vi "split.vi"(0 "object in":refnum<class "access_work.lvclass">, 1 "输入数据":string[][](array[string]), 2 "拆分大小":i32=1000, 5 "error in (no error)":errorcluster) -> (14 "object out":refnum<class "access_work.lvclass">, 15 "输出数组":string[][](array[string]), 16 "拆分数据":bool, 19 "error out":errorcluster)   [LabVIEW 2016, in "access_work.lvclass"]
uses:
  access_work.lvclass
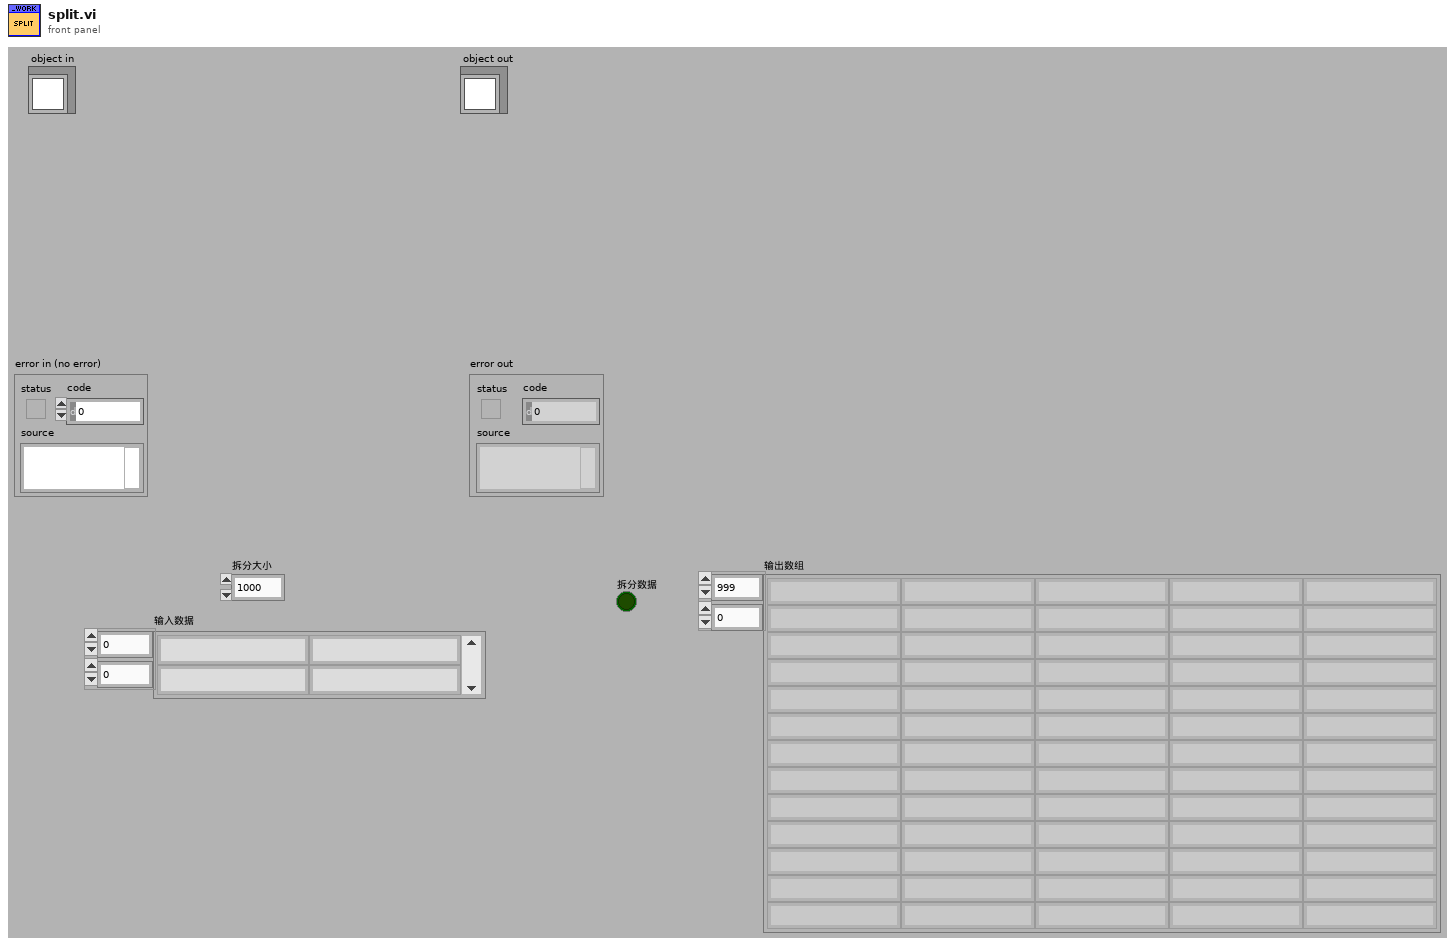
[diagram p1: front panel]
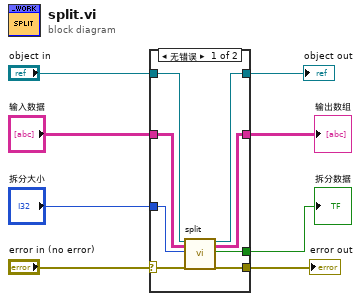
[diagram p0: block diagram]
diagram:
  n1 = case shown="无错误" "error in (no error)" {
    selector: "error in (no error)" -> [w10 w18]
    tunnel: [w9 w18] -> w7
    tunnel: [w13 w17] -> w5
    tunnel: "object in" -> [w16 w17]
    tunnel: "输入数据" -> [w15 _]
    tunnel: "拆分大小" -> [w14 _]
    tunnel: [w12 _] -> w2
    tunnel: [w11 _] -> w1
    frame No Error {
      n2 = call-dynamic "split.vi"("object in"=w16, "输入数据"=w15, "拆分大小"=w14, "error in (no error)"=w10) -> ("object out"=w13:refnum<class "access_work.lvclass">, "输出数组"=w11:string[][], "拆分数据"=w12:bool, "error out"=w9:errorcluster)  [unwired: 12 in]
    }
    frame Error {
    }
  }
  "error out" <- w7
  "object out" <- w5
  "输出数组" <- w1
  "拆分数据" <- w2
